vi "Parameter Analyzer Data.vi"() -> (0 "HP4155C Data":T1={"Configuration"={"Parameter Analyzer VISA Session"="COM1", "Sweeping Time Parameters"={"Integration Time"=0, "Short Integration Time (s)"=1.0, "Long Integration Time (s)"=0.0, "Wait Time Parameter"=1.0}, "Acquisition Mode"=enum."Sweeping Mode", "Status Polling Time (ms)"=1000, "Comment"="Test VI", "SMU 1 - Sweeping"={"Start / Offset"=0.0, "Stop / Ratio"=1.0, "Step \n(linear only)"=0.01, "Compliance"=0.1, "Power \nCompliance"=0.0, "Mode"=0, "Function"=0, "Sweep Mode"=FALSE}, "SMU 2 - Sweeping"={"Start / Offset"=0.0, "Stop / Ratio"=1.0, "Step \n(linear only)"=0.01, "Compliance"=0.1, "Power \nCompliance"=0.0, "Mode"=0, "Function"=0, "Sweep Mode"=FALSE}, "SMU 3 - Sweeping"={"Start / Offset"=0.0, "Stop / Ratio"=1.0, "Step \n(linear only)"=0.01, "Compliance"=0.1, "Power \nCompliance"=0.0, "Mode"=0, "Function"=0, "Sweep Mode"=FALSE}, "SMU 4 - Sweeping"={"Start / Offset"=0.0, "Stop / Ratio"=1.0, "Step \n(linear only)"=0.01, "Compliance"=0.1, "Power \nCompliance"=0.0, "Mode"=0, "Function"=0, "Sweep Mode"=FALSE}, "Sweep Spacing"=0, "Range"=0, "SMU1 - Sampling"={"Source"=10.0, "Compliance"=1e-05, "Mode"=0, "Function"=FALSE}, "SMU2 - Sampling"={"Source"=10.0, "Compliance"=1e-05, "Mode"=0, "Function"=FALSE}, "SMU3 - Sampling"={"Source"=10.0, "Compliance"=1e-05, "Mode"=0, "Function"=FALSE}, "SMU4 - Sampling"={"Source"=0.1, "Compliance"=60.0, "Mode"=0, "Function"=FALSE}, "Sampling Time Parameters"={"Initial Interval (s)"=0.1, "Number of Samples"=60, "Total Sampling Time (s)"=10.0, "Hold Time (s)"=0.0, "Sampling Mode"=0, "Sampling Time"=0}, "Stop Condition"={"Enable Delay (s)"=0.0, "Name"="", "Threshold"=0.0, "num. of events"=1, "Event"=0, "Stop Condition Enable"=FALSE}}, "Refnums"={"Status"=refnum, "Electrical Measurement"=refnum, "Plots"={"Plot List"=refnum, "Voltage Plot"=refnum, "Current Plot"=refnum, "IV Characteristic"=refnum, "dI/dV-V Characteristic"=refnum}, "HP Integration Time"=refnum, "VISA"=refnum, "Sweeping Time Parameters"=refnum, "Acquisition Mode"=refnum, "SMU 1 - Sweeping"=refnum, "SMU 2 - Sweeping"=refnum, "SMU 3 - Sweeping"=refnum, "SMU 4 - Sweeping"=refnum, "Sweep Spacing"=refnum, "Range"=refnum, "SMU1 - Sampling"=refnum, "SMU2 - Sampling"=refnum, "SMU3 - Sampling"=refnum, "SMU4 - Sampling"=refnum, "Sampling Time Parameters"=refnum, "Stop Condition"=refnum, "Instrument Status"=refnum}, "Initialization"={"Update Visa Session"=FALSE, "Configure Integration Time"=FALSE, "Configure Acquisition Mode"=FALSE, "Update Refnums"=FALSE}} {"Configuration"."Stop Condition"."Event" items=["Value > Threshold", "Value < Threshold", "| Value | > | Threshold |", "| Value | < | Threshold |"]; "Configuration"."Stop Condition"."Threshold" format="%^.2e"; "Configuration"."Stop Condition"."Enable Delay (s)" format="%.1f"; "Configuration"."Sampling Time Parameters"."Sampling Time" items=["Auto (linear only)", "No Limit", "Set Limit"]; "Configuration"."Sampling Time Parameters"."Sampling Mode" items=["Linear", "Log10", "Log25", "Log50", "Thinned Out"]; "Configuration"."Sampling Time Parameters"."Hold Time (s)" format="%.4f"; "Configuration"."Sampling Time Parameters"."Total Sampling Time (s)" format="%.1f"; "Configuration"."Sampling Time Parameters"."Initial Interval (s)" format="%^.3e"; "Configuration"."SMU 4 - Sweeping"."Function" items=["Disabled", "Var 1", "Var 2", "Var 1'", "Constant"]; "Configuration"."SMU 4 - Sweeping"."Mode" items=["V", "I", "V pulse", "I  pulse", "Common"]; "Configuration"."SMU 4 - Sweeping"."Power \nCompliance" format="%^.2e"; "Configuration"."SMU 4 - Sweeping"."Compliance" format="%^.2e"; "Configuration"."SMU 4 - Sweeping"."Step \n(linear only)" format="%^.4e"; "Configuration"."SMU 4 - Sweeping"."Stop / Ratio" format="%^.4e"; "Configuration"."SMU 4 - Sweeping"."Start / Offset" format="%^.4e"; "Configuration"."SMU 3 - Sweeping"."Function" items=["Disabled", "Var 1", "Var 2", "Var 1'", "Constant"]; "Configuration"."SMU 3 - Sweeping"."Mode" items=["V", "I", "V pulse", "I  pulse", "Common"]; "Configuration"."SMU 3 - Sweeping"."Power \nCompliance" format="%^.2e"; "Configuration"."SMU 3 - Sweeping"."Compliance" format="%^.2e"; "Configuration"."SMU 3 - Sweeping"."Step \n(linear only)" format="%^.4e"; "Configuration"."SMU 3 - Sweeping"."Stop / Ratio" format="%^.4e"; "Configuration"."SMU 3 - Sweeping"."Start / Offset" format="%^.4e"; "Configuration"."SMU 2 - Sweeping"."Function" items=["Disabled", "Var 1", "Var 2", "Var 1'", "Constant"]; "Configuration"."SMU 2 - Sweeping"."Mode" items=["V", "I", "V pulse", "I  pulse", "Common"]; "Configuration"."SMU 2 - Sweeping"."Power \nCompliance" format="%^.2e"; "Configuration"."SMU 2 - Sweeping"."Compliance" format="%^.2e"; "Configuration"."SMU 2 - Sweeping"."Step \n(linear only)" format="%^.4e"; "Configuration"."SMU 2 - Sweeping"."Stop / Ratio" format="%^.4e"; "Configuration"."SMU 2 - Sweeping"."Start / Offset" format="%^.4e"; "Configuration"."SMU 1 - Sweeping"."Function" items=["Disabled", "Var 1", "Var 2", "Var 1'", "Constant"]; "Configuration"."SMU 1 - Sweeping"."Mode" items=["V", "I", "V pulse", "I  pulse", "Common"]; "Configuration"."SMU 1 - Sweeping"."Power \nCompliance" format="%^.2e"; "Configuration"."SMU 1 - Sweeping"."Compliance" format="%^.2e"; "Configuration"."SMU 1 - Sweeping"."Step \n(linear only)" format="%^.4e"; "Configuration"."SMU 1 - Sweeping"."Stop / Ratio" format="%^.4e"; "Configuration"."SMU 1 - Sweeping"."Start / Offset" format="%^.4e"; "Configuration"."Sweeping Time Parameters"."Long Integration Time (s)" scale=0.02..2.0; "Configuration"."Sweeping Time Parameters"."Short Integration Time (s)" scale=8e-05..0.00192; "Configuration"."Sweeping Time Parameters"."Integration Time" items=["Short", "Long"]; "Configuration"."Sweeping Time Parameters"."Wait Time Parameter" format="%.1f"; "Configuration"."SMU4 - Sampling"."Mode" items=["V", "I", "Common"]; "Configuration"."SMU4 - Sampling"."Compliance" format="%^.2e"; "Configuration"."SMU4 - Sampling"."Source" format="%^.3e"; "Configuration"."SMU3 - Sampling"."Mode" items=["V", "I", "Common"]; "Configuration"."SMU3 - Sampling"."Compliance" format="%^.2e"; "Configuration"."SMU3 - Sampling"."Source" format="%^.3e"; "Configuration"."SMU2 - Sampling"."Mode" items=["V", "I", "Common"]; "Configuration"."SMU2 - Sampling"."Compliance" format="%^.2e"; "Configuration"."SMU2 - Sampling"."Source" format="%^.3e"; "Configuration"."SMU1 - Sampling"."Mode" items=["V", "I", "Common"]; "Configuration"."SMU1 - Sampling"."Compliance" format="%^.2e"; "Configuration"."SMU1 - Sampling"."Source" format="%^.3e"; "Configuration"."Range" items=["auto", "fixed", "limited"]; "Configuration"."Sweep Spacing" items=["linear", "log 10", "log 25", "log 50"]})   [LabVIEW 2014]
uses:
  Parameter Analyzer Data.ctl
  Parameter Analyzer Config.ctl
  Parameter Analyzer Integration Parameters.ctl
  Parameter Analyzer SMU Sweeping.ctl
  Parameter Analyzer Sweep Spacing.ctl
  Parameter Analyzer SMU Range.ctl
  Parameter Analyzer SMU Sampling.ctl
  Parameter Analyzer Sampling Parameters.ctl
  Parameter Analyzer Stop Sampling Conditions.ctl
  Parameter Analyzer Refnums.ctl
  Measurements/Plot Data/Electrical Data Plot Refnums.ctl
  Parameter Analyzer Initialization.ctl
panel:
  # "LICENSED MATERIALS – PROPERTY OF IBM\nCopyright IBM Corp. 2016,\nALL RIGHTS RESERVED"
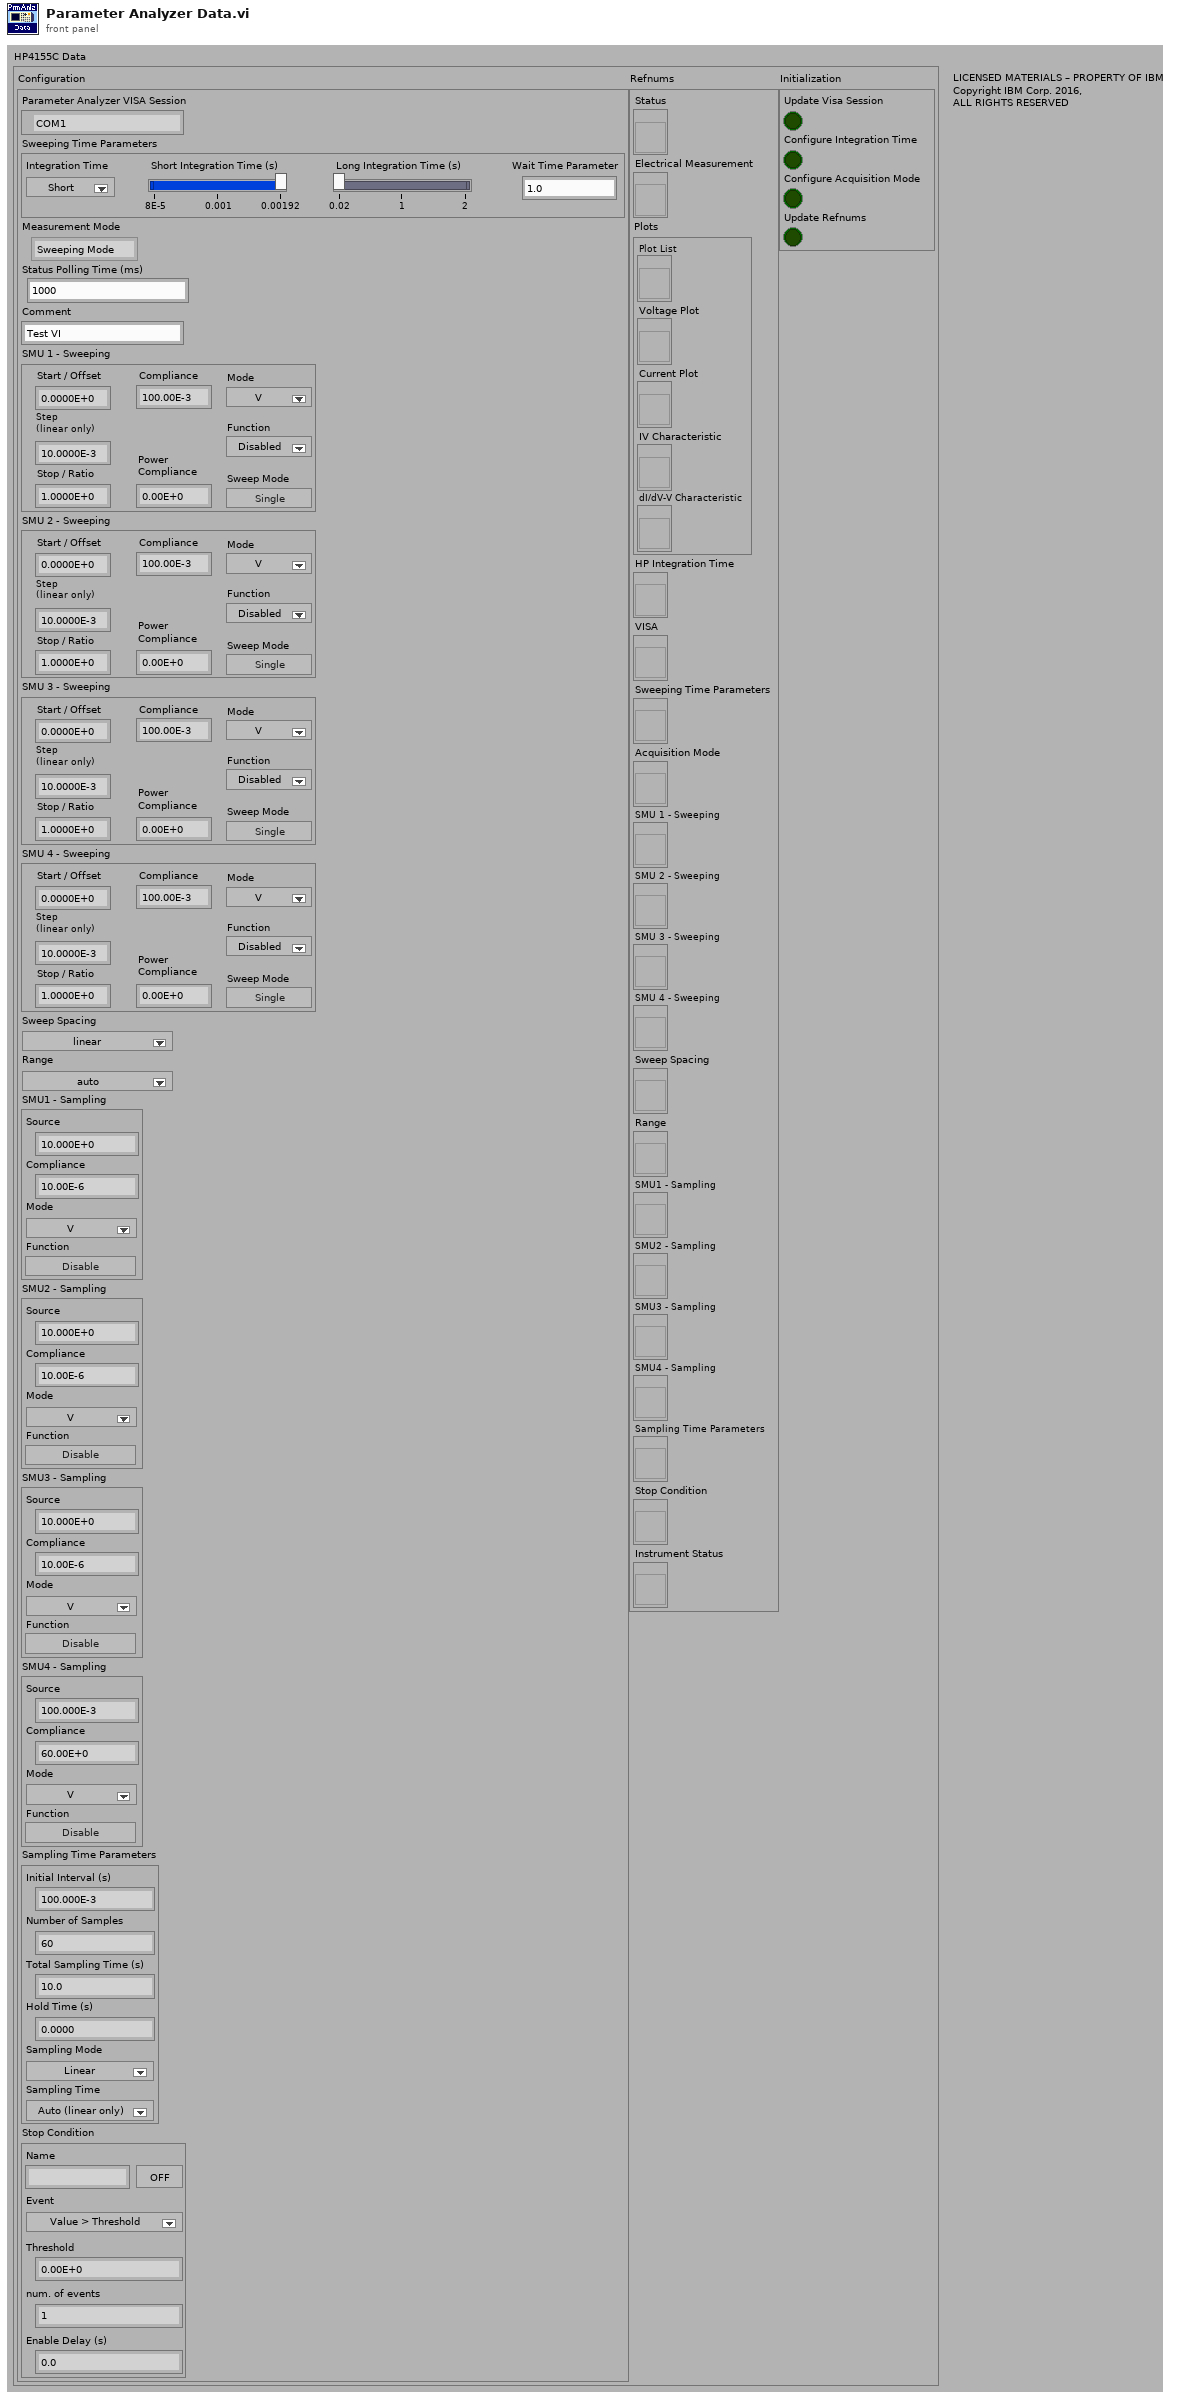
[diagram p1: front panel]
types:
  T1 = typedef "Parameter Analyzer Data.ctl" = cluster{"Configuration":T2, "Refnums":T10, "Initialization":T12}
  T2 = typedef "Parameter Analyzer Config.ctl" = cluster{"Parameter Analyzer VISA Session":refnum<visa-resource-name>, "Sweeping Time Parameters":T3, "Acquisition Mode":enum32{"Sweeping Mode", "Sampling Mode"}, "Status Polling Time (ms)":u32, "Comment":string, "SMU 1 - Sweeping":T4, "SMU 2 - Sweeping":T4, "SMU 3 - Sweeping":T4, "SMU 4 - Sweeping":T4, "Sweep Spacing":T5, "Range":T6, "SMU1 - Sampling":T7, "SMU2 - Sampling":T7, "SMU3 - Sampling":T7, "SMU4 - Sampling":T7, "Sampling Time Parameters":T8, "Stop Condition":T9}
  T3 = typedef "Parameter Analyzer Integration Parameters.ctl" = cluster{"Integration Time":u32, "Short Integration Time (s)":dbl, "Long Integration Time (s)":dbl, "Wait Time Parameter":dbl}
  T4 = typedef "Parameter Analyzer SMU Sweeping.ctl" = cluster{"Start / Offset":dbl, "Stop / Ratio":dbl, "Step \n(linear only)":dbl, "Compliance":dbl, "Power \nCompliance":dbl, "Mode":u32, "Function":i32, "Sweep Mode":bool}
  T5 = typedef "Parameter Analyzer Sweep Spacing.ctl" = u16
  T6 = typedef "Parameter Analyzer SMU Range.ctl" = u16
  T7 = typedef "Parameter Analyzer SMU Sampling.ctl" = cluster{"Source":dbl, "Compliance":dbl, "Mode":u32, "Function":bool}
  T8 = typedef "Parameter Analyzer Sampling Parameters.ctl" = cluster{"Initial Interval (s)":dbl, "Number of Samples":i32, "Total Sampling Time (s)":dbl, "Hold Time (s)":dbl, "Sampling Mode":i32, "Sampling Time":i32}
  T9 = typedef "Parameter Analyzer Stop Sampling Conditions.ctl" = cluster{"Enable Delay (s)":dbl, "Name":string, "Threshold":dbl, "num. of events":i32, "Event":i32, "Stop Condition Enable":bool}
  T10 = typedef "Parameter Analyzer Refnums.ctl" = cluster{"Status":refnum<vi>, "Electrical Measurement":refnum<vi>, "Plots":T11, "HP Integration Time":refnum<vi>, "VISA":refnum<vi>, "Sweeping Time Parameters":refnum<vi>, "Acquisition Mode":refnum<vi>, "SMU 1 - Sweeping":refnum<vi>, "SMU 2 - Sweeping":refnum<vi>, "SMU 3 - Sweeping":refnum<vi>, "SMU 4 - Sweeping":refnum<vi>, "Sweep Spacing":refnum<vi>, "Range":refnum<vi>, "SMU1 - Sampling":refnum<vi>, "SMU2 - Sampling":refnum<vi>, "SMU3 - Sampling":refnum<vi>, "SMU4 - Sampling":refnum<vi>, "Sampling Time Parameters":refnum<vi>, "Stop Condition":refnum<vi>, "Instrument Status":refnum<vi>}
  T11 = typedef "Electrical Data Plot Refnums.ctl" = cluster{"Plot List":refnum<vi>, "Voltage Plot":refnum<vi>, "Current Plot":refnum<vi>, "IV Characteristic":refnum<vi>, "dI/dV-V Characteristic":refnum<vi>}
  T12 = typedef "Parameter Analyzer Initialization.ctl" = cluster{"Update Visa Session":bool, "Configure Integration Time":bool, "Configure Acquisition Mode":bool, "Update Refnums":bool}
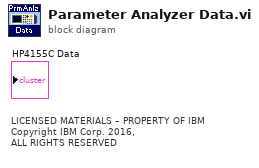
[diagram p0: block diagram]
diagram:
  # "LICENSED MATERIALS – PROPERTY OF IBM\nCopyright IBM Corp. 2016,\nALL RIGHTS RESERVED"
